vi "Polar To Complex - R,RM.vi"(1 "Argument Q":T1, 2 "Modulus Scalar  r":dbl) -> (0 "Complex Matrix r*e^iQ":T2)   [LabVIEW 2018, in "NI_Matrix.lvlib"]
doc: "Creates a complex number from two values in polar notation."
uses:
  NI_Matrix.lvlib
  ComplexMatrix.ctl
  RealMatrix.ctl
  Matrix To Array - RM.vi
  Array To Matrix - CA2.vi
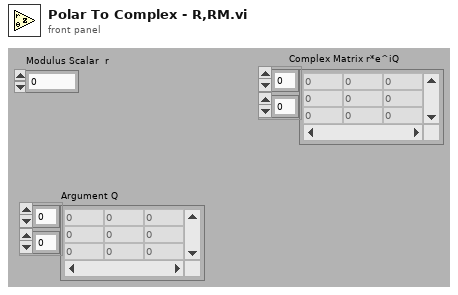
[diagram p1: front panel]
types:
  T1 = typedef "NI_Matrix.lvlib/RealMatrix.ctl" = dbl[][]
  T2 = typedef "NI_Matrix.lvlib/ComplexMatrix.ctl" = cdb[][]
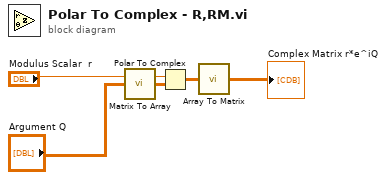
[diagram p0: block diagram]
diagram:
  n1 = call-poly "Matrix To Array.vi"("Real Matrix"="Argument Q") -> ("Real 2D Array"=w4:dbl[][])
  n2 = Polar To Complex(1:w4, 2:"Modulus Scalar  r") -> (0:w2:cdb[][])
  n3 = call-poly "Array To Matrix.vi"("Complex 2D Array"=w2) -> ("Complex Matrix"=→"Complex Matrix r*e^iQ":T2)
